vi "NewLot.vi"(7 "FilePath":path, 8 "error in (no error)":errorcluster, 9 "Type":string, 10 "Wafer ID":string, 11 "LotData in":refnum<class "LotData.lvclass">) -> (0 "error out":errorcluster, 3 "LotData out":refnum<class "LotData.lvclass">)   [LabVIEW 2012, in "LotData.lvclass"]
uses:
  LotData.lvclass
  Controls/TestData.ctl
  Controls/LotData_Current.ctl
  LotData.lvclass/LotData.ctl
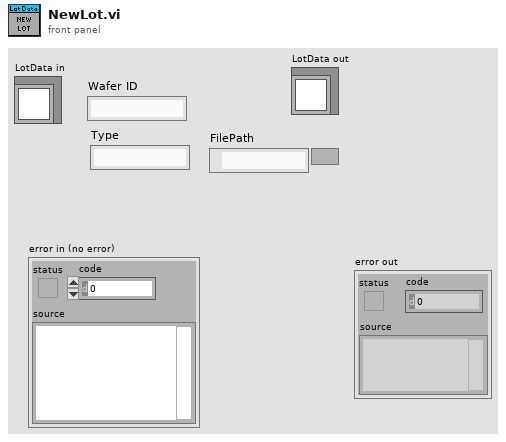
[diagram p1: front panel]
types:
  T1 = cluster{"Area":string, "Wavelength":dbl[], "EL Spectrum":dbl[]}
  T2 = typedef "TestData.ctl" = cluster{"20mA Data":cluster{"Area":string, "Current,mA":dbl, "Power":dbl, "WL":dbl, "Voltage":dbl, "Knee Current":dbl, "Reverse":dbl}, "50mA Data":cluster{"Area":string, "Current,mA":dbl, "Power":dbl, "WL":dbl, "Voltage":dbl}}
  T3 = typedef "LotData.lvclass/LotData_Current.ctl" = cluster{"area":i32, "Data":cluster{"wl":dbl, "power":dbl, "voltage":dbl, "knee":dbl, "reverse":dbl}}
  T4 = cluster{"Area":string, "Current,mA":dbl, "Power":dbl, "WL":dbl, "Voltage":dbl, "Knee Current":dbl, "Reverse":dbl}
  T5 = cluster{"Area":string, "Current,mA":dbl, "Power":dbl, "WL":dbl, "Voltage":dbl}
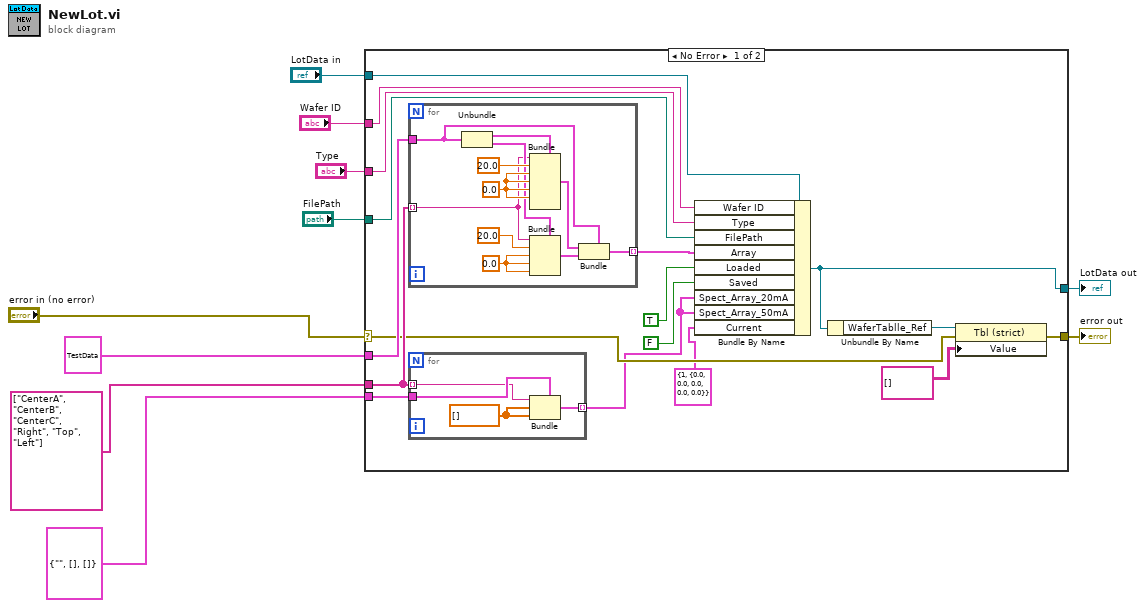
[diagram p0: block diagram]
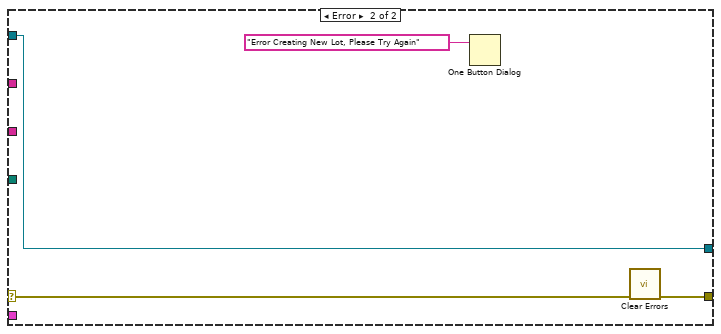
[diagram p2: hidden frame]
diagram:
  n1 = case shown="No Error" "error in (no error)" {
    selector: "error in (no error)" -> [w15 w44]
    tunnel: [w18 w43] -> w9
    tunnel: "LotData in" -> [w11 w46]
    tunnel: "Wafer ID" -> [w27 _]
    tunnel: "Type" -> [w14 _]
    tunnel: "FilePath" -> [w26 _]
    tunnel: T2 {"20mA Data"={"Area"="", "Current,mA"=0.0, "Power"=0.0, "WL"=0.0, "Voltage"=0.0, "Knee Current"=0.0, "Reverse"=0.0}, "50mA Data"={"Area"="", "Current,mA"=0.0, "Power"=0.0, "WL"=0.0, "Voltage"=0.0}} ("TestData") -> [w25 _]
    tunnel: string[] ["CenterA", "CenterB", "CenterC", "Right", "Top", "Left"] -> [w17 _]
    tunnel: [w19 w46] -> w4
    tunnel: T1 {"Area"="", "Wavelength"=[], "EL Spectrum"=[]} ("Spect") -> [w16 _]
    frame No Error {
      n2 = for {
        tunnel: w25 -> [w35]
        tunnel: w17 -> [w36] mode=indexing
        tunnel: [w32] -> w24 mode=indexing
        w39 = 0.0 ("Power")
        w40 = 0.0 ("Power")
        n3 = Unbundle(w35) -> ("20mA Data"=w42:T4, "50mA Data"=w37:T5)
        n4 = Bundle(cluster=w42, "Area"=w36, "Current,mA"=20.0, "Power"=w40, "WL"=w40, "Voltage"=w40, "Knee Current"=w40) -> (w34:T4)  [unwired: 1 in]
        n5 = Bundle(cluster=w37, "Area"=w36, "Current,mA"=20.0, "Power"=w39, "WL"=w39, "Voltage"=w39) -> (w33:T5)
        n6 = Bundle(cluster=w35, "20mA Data"=w34, "50mA Data"=w33) -> (w32:T2)
      }
      n7 = for {
        tunnel: w17 -> [w30] mode=indexing
        tunnel: w16 -> [w31]
        tunnel: [w28] -> w13 mode=indexing
        w29 = dbl[] [] ("Wavelength")
        n8 = Bundle(cluster=w31, "Area"=w30, "Wavelength"=w29, "EL Spectrum"=w29) -> (w28:T1)
      }
      n9 = Bundle By Name(cluster=w11, "Wafer ID"=w27, "Type"=w14, "FilePath"=w26, "Array"=w24, "Loaded"=TRUE, "Saved"=FALSE, "Spect_Array_20mA"=w13, "Spect_Array_50mA"=w13, "Current"=T3 {"area"=1, "Data"={"wl"=0.0, "power"=0.0, "voltage"=0.0, "knee"=0.0, "reverse"=0.0}}) -> (w19:refnum<class "LotData.lvclass">)
      n10 = Unbundle By Name(w19) -> ("WaferTablle_Ref"=w20:refnum<vi>)
      n11 = property class="Tbl (strict)"(reference=w20, error in=w15, "Value"=string[][] []) -> (error out=w18:errorcluster)  [unwired: 1 out]
    }
    frame Error {
      n12 = One Button Dialog(message="Error Creating New Lot, Please Try Again") -> ()  [unwired: 1 in, 1 out]
      n13 = call <vilib>:"Clear Errors.vi"("error in (no error)"=w44) -> ("error out"=w43:errorcluster)  [unwired: 6 in]
    }
  }
  "error out" <- w9
  "LotData out" <- w4
